vi "TemperatureLimit.vi"() -> ()   [LabVIEW 2025]
panel:
  in  "stop":bool
  out "Limit Exceeded?":bool
  in  "Lower limit":dbl
  in  "Upper Limit":dbl
  out "Temperature chart":T1(graph)
  in  "Temp C":dbl
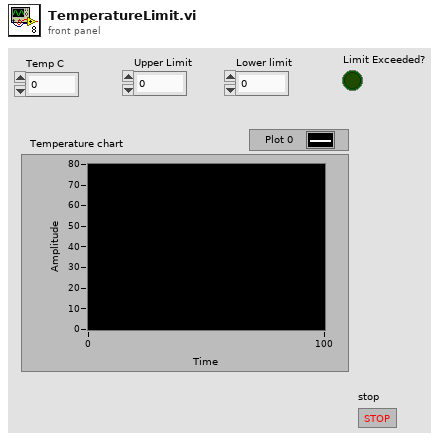
[diagram p1: front panel]
types:
  T1 = cluster{"Temp C":dbl, "Upper Limit":dbl, "Lower limit":dbl}
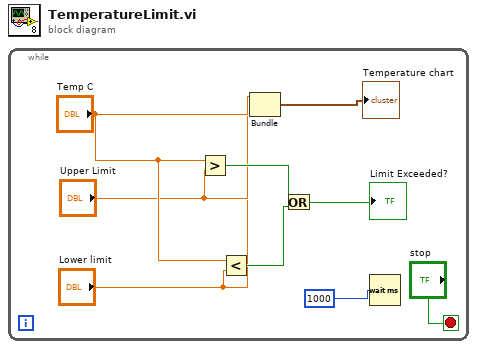
[diagram p0: block diagram]
diagram:
  n1 = while {
    stop <- "stop" stop-if-true
    n2 = Greater?(x="Temp C", y="Upper Limit") -> (0:w9:bool)
    n3 = Less?(x="Temp C", y="Lower limit") -> (x < y?=w8:bool)
    n4 = Bundle("Temp C"="Temp C", "Upper Limit"="Upper Limit", "Lower limit"="Lower limit") -> (→"Temperature chart":T1)  [unwired: 1 in]
    n5 = Or(x=w9, y=w8) -> (x .or. y?=→"Limit Exceeded?":bool)
    n6 = Wait (ms)(milliseconds to wait=1000) -> ()  [unwired: 1 out]
  }
